vi "Analyze Data.vi"(8 "error in":errorcluster, 11 "tCRD in":refnum<class "Aircraft OPCCRD.lvclass">) -> (0 "error out":errorcluster, 3 "tCRD out":refnum<class "Aircraft OPCCRD.lvclass">)   [LabVIEW 2015, in "Aircraft OPCCRD.lvclass"]
doc: "Analyze Data takes the stored ringdown data (1000 shots per cell) and:\n1) Calculates the ringdown decay constant tau\n2) Averages tau0 data as necessary\n3) Corrects the tau data for Rayleigh scattering\n4) Stores a 1-D array of taus returned on a 1 kHz basis (8k taus) if a jump drive (U:) is connected\n5) Flattens the data into a string and stuffs the string into the <b>data</b> shared variable for display on the UI.\n\nThis VI will not be called if the data is not \"good\" (that is, if an error was thrown in the <B>Get Data</B> routine. If an error is thrown while the data is being retrieved, then the data will not be sent to the UI."
uses:
  Aircraft OPCCRD.lvclass
  Reusable/CRDS/Main/CRDS.lvclass/CRDS.ctl
  Reusable/Instrument/Instrument.lvclass/Instrument.ctl
  Aircraft OPCCRD.lvclass/Aircraft OPCCRD.ctl
  Reusable/CRDS/Cell/CRDS Cell.lvclass/CRDS Cell.ctl
  Reusable/CRDS/Data/Cell/CRDS Cell Data.lvclass/CRDS Cell Data.ctl
  <vilib>/Analysis/baseanly.llb/Matrix Type of Inverse Matrix.ctl
  Reusable/File IO/Class/File Observer.lvclass/File Observer.ctl
  <vilib>/Analysis/7linalg.llb/Solve Linear Equations (single right hand).vi
  <vilib>/Analysis/baseanly.llb/Mean (DBL).vi
  Reusable/File IO/Class/Read File Ref.vi
  Reusable/CRDS/Data/Cell/Read extParam.vi
  Reusable/CRDS/Data/Cell/Write FitCoeff.vi
  Reusable/CRDS/Data/Cell/Write extParam.vi
  Reusable/CRDS/Cell/Write Data.vi
  Accessors/Write tau Obs.vi
  Reusable/CRDS/Main/Read Laser Data.vi
  Reusable/Instrument/Read Log Session.vi
  Reusable/CRDS/Main/Read CRD RD Data Obs.vi
  Reusable/CRDS/Main/Write CRD RD Data Obs.vi
  Reusable/CRDS/Main/Read writeRDs.vi
  <vilib>/Analysis/baseanly.llb/Solve Linear Equations By Cholesky.vi
  <vilib>/Analysis/baseanly.llb/Real Matrix to Compact Array.vi
  <vilib>/Analysis/baseanly.llb/Real Compact Tri-Matrix Linear Eqs.vi
  Reusable/CRDS/Main/Read Cells.vi
  Reusable/CRDS/Main/Read goodData.vi
  Reusable/CRDS/Data/Main/Read filter.vi
  Reusable/Data/Read measTime.vi
  Reusable/CRDS/Cell/Read dt.vi
  <vilib>/Analysis/7linalg.llb/Solve Linear Eqs (General).vi
  <vilib>/Analysis/7linalg.llb/Solve Linear Eqs (Gen, single right hand).vi
  Reusable/CRDS/Data/Cell/Write Ringdowns.vi
  Reusable/CRDS/Main/Write Cells.vi
  Reusable/CRDS/Main/Write Data.vi
  Reusable/CRDS/Cell/CRDS Cell.lvclass
  Reusable/CRDS/Data/Main/CRDS Data.lvclass
  <userlib>/_Session Fwk/Session - Root.lvclass
  Reusable/CRDS/Data/Cell/CRDS Cell Data.lvclass
  Reusable/File IO/Class/File Observer.lvclass
  <vilib>/Analysis/NI_AALPro.lvlib
  <vilib>/Analysis/NI_AALBase.lvlib
  Reusable/Session Log/System Log.lvclass
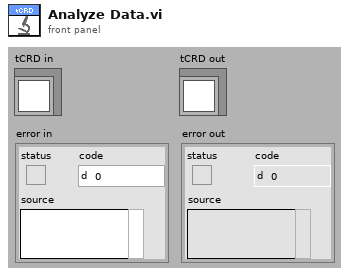
[diagram p1: front panel]
types:
  T1 = typedef "NI_AALBase.lvlib/Matrix Type of Inverse Matrix.ctl" = enum32{"General", "Positive Definite", "Lower Triangular", "Upper Triangular"}
  T2 = typedef "Session - Root.lvclass/Session Handle.ctl" = refnum<data-value>
  T3 = typedef "extparam.ctl" = cluster{"Tau":sgl, "Tau0cor":sgl, "ext":sgl, "extCorr":sgl, "stdevTau":sgl, "eTau":sgl, "taucorr":sgl, "Tau0":sgl, "max":sgl}
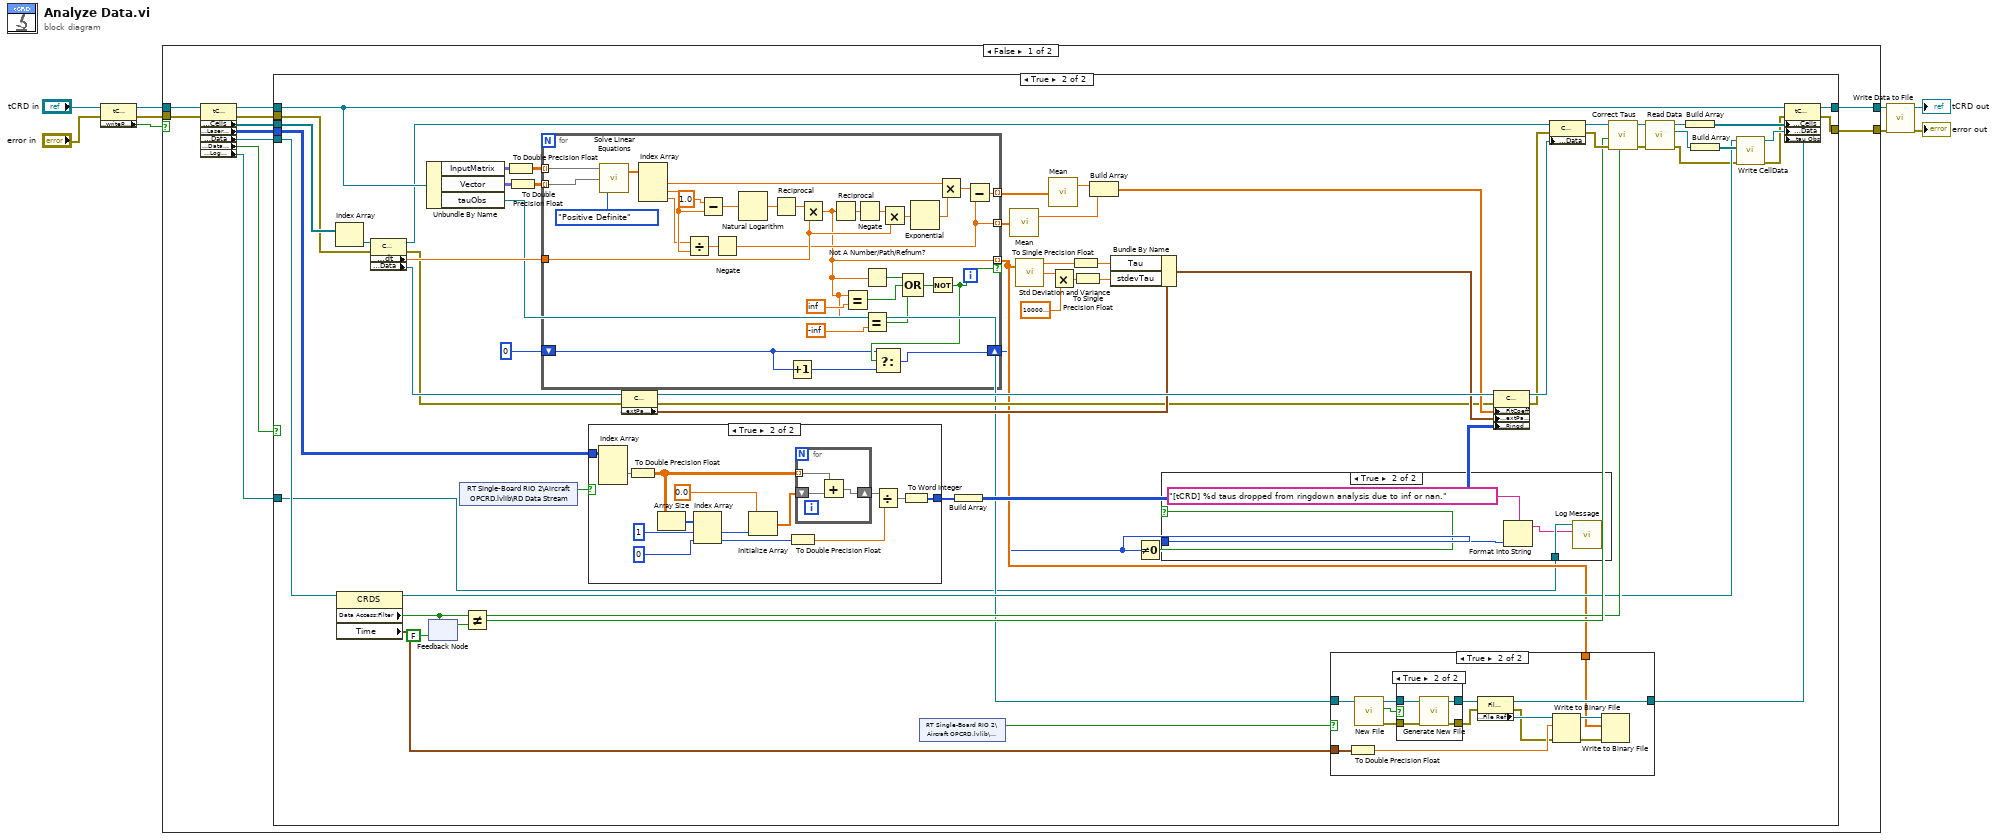
[diagram p0: block diagram]
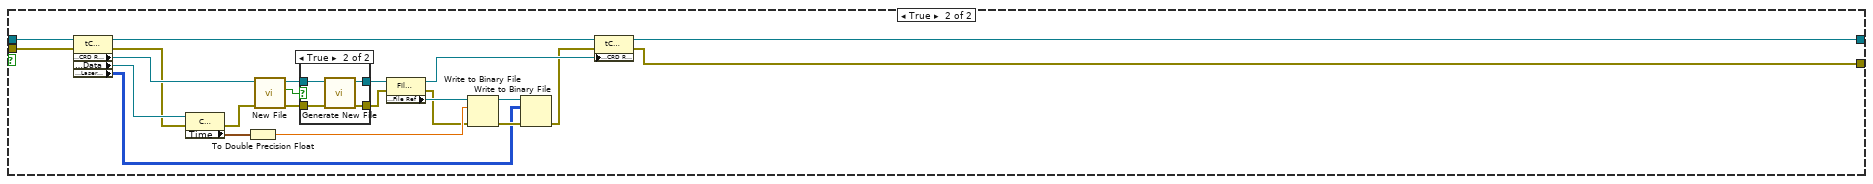
[diagram p7: hidden frame]
diagram:
  n1 = property class="tCRD"(reference="tCRD in", error in="error in") -> (reference out=w4:refnum<class "Aircraft OPCCRD.lvclass">, error out=w3:errorcluster, "Accessors:writeRDs"=w1:bool)
  n2 = case shown="False" w1 {
    tunnel: w3 -> [w20 w176]
    tunnel: [w18 w179] -> w9
    tunnel: [w17 w178] -> w7
    tunnel: w4 -> [w16 w177]
    frame False {
      n3 = property class="tCRD"(reference=w16, error in=w20) -> (reference out=w15:refnum<class "Aircraft OPCCRD.lvclass">, error out=w11:errorcluster, "Data Access:Cells"=w19:refnum<class "CRDS Cell.lvclass">[], "Data Access:Laser Data"=w13:i16[][][], "Data Access:Data"=w14:refnum<class "CRDS Data.lvclass">, "Data Access:Data Ready?"=w12:bool, "Accessors:Log Session"=w10:T2)
      n4 = case shown="True" w12 {
        tunnel: w19 -> [_ w83]
        tunnel: [w22 w63] -> w18
        tunnel: [w21 w62] -> w17
        tunnel: w15 -> [w22 w48]
        tunnel: w14 -> [_ w47]
        tunnel: w13 -> [_ w38]
        tunnel: w11 -> [w21 w34]
        tunnel: w10 -> [_ w23]
        frame False {
        }
        frame True {
          n5 = Index Array(array=w83) -> (element=w76:refnum<class "CRDS Cell.lvclass">)  [unwired: 1 in]
          n6 = property class="CRDS"(reference=w47) -> (reference out=w46:refnum<class "CRDS Data.lvclass">, "Data Access:Filter"=w70:bool, "Time"=w29:timestamp)  [unwired: 1 in, 1 out]
          n7 = property class="CRDS Cell"(reference=w76, error in=w34) -> (reference out=w45:refnum<class "CRDS Cell.lvclass">, error out=w33:errorcluster, "Data Access:dt"=w64:dbl, "Data Access:Data"=w82:refnum<class "CRDS Cell Data.lvclass">)
          n8 = Unbundle By Name(w48) -> ("InputMatrix"=w61:fxp<+/-,64,64>[][][], "Vector"=w59:fxp<+/-,64,64>[][], "tauObs"=w31:refnum<class "File Observer.lvclass">)
          n9 = feedback #1(FALSE ("filter")) -> (w56:bool)
          n10 = feedback-in #1(w70) -> ()
          n11 = shared-variable "RT Single-Board RIO 2\\Aircraft OPCRD.lvlib\\RD Data Stream"() -> (w49:bool)  [unwired: 1 in, 1 out]
          n12 = Not Equal?(x=w70, y=w56) -> (x != y?=w71:bool)
          n13 = To Double Precision Float(number=w61) -> (double precision float=w60:dbl[][][])
          n14 = To Double Precision Float(number=w59) -> (double precision float=w58:dbl[][])
          n15 = for {
            tunnel: w58 -> [w141] mode=indexing
            tunnel: w64 -> [w140]
            tunnel: [w134] -> w28 mode=indexing if=w129
            tunnel: w60 -> [w139] mode=indexing
            tunnel: [w138] -> w54 mode=indexing
            tunnel: [w137] -> w53 mode=indexing
            shift-right: [w126] -> w25
            shift-left: 0 -> [w128]
            n16 = call-poly <vilib>:"Solve Linear Equations.vi"("matrix type"=Matrix_Type_of_Inverse_Matrix."Positive Definite", "Known Vector"=w141, "Input Matrix"=w139) -> ("Solution Vector"=w155:dbl[])  [unwired: 1 out]
            n17 = Index Array(array=w155) -> (element #1=w144:dbl, element #2=w143:dbl, element #3=w142:dbl)  [unwired: 3 in]
            n18 = Divide(x=w142, y=w143) -> (x/y=w150:dbl)
            n19 = Subtract(x=1.0, y=w143) -> (x-y=w153:dbl)
            n20 = Negate(x=w150) -> (-x=w138:dbl)
            n21 = Natural Logarithm(1:w153) -> (0:w152:dbl)
            n22 = Reciprocal(x=w152) -> (1/x=w151:dbl)
            n23 = Increment(x=w128) -> (x+1=w127:i32)
            n24 = Multiply(x=w151, y=w140) -> (x*y=w134:dbl)
            n25 = Reciprocal ("beta")(x=w134) -> (1/x=w149:dbl)
            n26 = Equal?(x=w134, y=inf) -> (x = y?=w132:bool)
            n27 = Negate(x=w149) -> (-x=w148:dbl)
            n28 = Not A Number/Path/Refnum?(number/path/refnum=w134) -> (NaN/Path/Refnum?=w133:bool)
            n29 = Equal?(x=w134, y=-inf) -> (x = y?=w130:bool)
            n30 = Multiply(x=w148, y=w140) -> (x*y=w147:dbl)
            n31 = Compound Arithmetic op=OR(w133, w132, w130) -> (w131:bool)
            n32 = Exponential(1:w147) -> (0:w145:dbl)
            n33 = Not(x=w131) -> (.not. x?=w129:bool)
            n34 = Select(t=w128, s=w129, f=w127) -> (s? t:f=w126:i32)
            n35 = Multiply(x=w144, y=w145) -> (x*y=w146:dbl)
            n36 = Subtract(x=w146, y=w138) -> (x-y=w137:dbl)
          }
          n37 = case shown="True" w49 {
            tunnel: [_ w121] -> w57
            tunnel: w38 -> [_ w115]
            frame False {
            }
            frame True {
              n38 = Index Array(array=w115) -> (element=w119:i16[][])  [unwired: 3 in]
              n39 = To Double Precision Float(number=w119) -> (double precision float=w113:dbl[][])
              n40 = Array Size(array=w113) -> (size(s)=w116:i32[])
              n41 = Index Array(array=w116, index #1=1 ("index"), index #2=0 ("index")) -> (element #1=w118:i32, element #2=w109:i32)
              n42 = Initialize Array(0.0 ("element"), w118) -> (w114:dbl[])
              n43 = To Double Precision Float(number=w109) -> (double precision float=w112:dbl)
              n44 = for {
                shift-right: [w123] -> w120
                shift-left: w114 -> [w124]
                tunnel: w113 -> [w125] mode=indexing
                n45 = Add(x=w125, y=w124) -> (x+y=w123:dbl[])
              }
              n46 = Divide(x=w120, y=w112) -> (x/y=w122:dbl[])
              n47 = To Word Integer(number=w122) -> (16bit integer=w121:i16[])
            }
          }
          n48 = property class="CRDS Cell"(reference=w82, error in=w33) -> (reference out=w81:refnum<class "CRDS Cell Data.lvclass">, error out=w32:errorcluster, "Data Access:extParam"=w80:T3)
          n49 = shared-variable "RT Single-Board RIO 2\\Aircraft OPCRD.lvlib\\WriteTau"() -> (w27:bool)  [unwired: 1 in, 1 out]
          n50 = Build Array(w57) -> (w79:i16[][])
          n51 = call-poly <vilib>:"Mean.vi"("X"=w54) -> ("mean"=w51:dbl)  [unwired: 1 out]
          n52 = call <vilib>:"Std Deviation and Variance.vi"("X"=w28) -> ("mean"=w42:dbl, "standard deviation"=w78:dbl)  [unwired: 1 in, 1 out]
          n53 = call-poly <vilib>:"Mean.vi"("X"=w53) -> ("mean"=w52:dbl)  [unwired: 1 out]
          n54 = Multiply(x=w78, y=1000000.0 ("stdevTau")) -> (x*y=w44:dbl)
          n55 = To Single Precision Float(number=w42) -> (single precision float=w41:sgl)
          n56 = To Single Precision Float(number=w44) -> (single precision float=w43:sgl)
          n57 = Build Array(w52, w51) -> (w39:dbl[])
          n58 = Bundle By Name(cluster=w80, "Tau"=w41, "stdevTau"=w43) -> (w40:T3)
          n59 = Not Equal To 0?(x=w25) -> (x != 0?=w24:bool)
          n60 = case shown="True" w24 {
            tunnel: w25 -> [_ w87]
            tunnel: w23 -> [_ w86]
            frame False {
            }
            frame True {
              n61 = Format Into String(format string="[tCRD] %d taus dropped from ringdown analysis due to inf or nan.", w87) -> (resulting string=w85:string)  [unwired: 2 in, 1 out]
              n62 = call "Log Message.vi"("MSG In"=w85, "session in"=w86) -> ()  [unwired: 8 in, 2 out]
            }
          }
          n63 = case shown="True" w27 {
            tunnel: w31 -> [w88 w92]
            tunnel: [w88 w91] -> w30
            tunnel: w29 -> [_ w90]
            tunnel: w28 -> [_ w89]
            frame False {
            }
            frame True {
              n64 = To Double Precision Float(number=w90) -> (double precision float=w96:dbl)
              n65 = call-dynamic "New File.vi"("File Observer in"=w92) -> ("error out"=w102:errorcluster, "Exceeded"=w101:bool, "File Observer out"=w100:refnum<class "File Observer.lvclass">)  [unwired: 8 in]
              n66 = case shown="True" w101 {
                tunnel: w100 -> [w104 w108]
                tunnel: [w104 w107] -> w99
                tunnel: w102 -> [w103 w106]
                tunnel: [w103 w105] -> w94
                frame False {
                }
                frame True {
                  n67 = call-dynamic "Generate New File.vi"("error in"=w106, "File Obs in"=w108) -> ("error out"=w105:errorcluster, "File Obs out"=w107:refnum<class "File Observer.lvclass">)  [unwired: 7 in, 1 out]
                }
              }
              n68 = property class="File Obs"(reference=w99, error in=w94) -> (reference out=w91:refnum<class "File Observer.lvclass">, error out=w93:errorcluster, "Data Access:File Ref"=w98:refnum<file>)
              n69 = Write to Binary File(file (use dialog)=w98, data=w96, error in=w93) -> (refnum out=w97:refnum<file>, error out=w95:errorcluster)  [unwired: 3 in, 1 out]
              n70 = Write to Binary File(file (use dialog)=w97, data=w89, error in=w95) -> ()  [unwired: 3 in, 3 out]
            }
          }
          n71 = property class="CRDS Cell"(reference=w81, error in=w32, "Accessors:FitCoeff"=w39, "Data Access:extParam"=w40, "Data Access:Ringdowns"=w79) -> (reference out=w50:refnum<class "CRDS Cell Data.lvclass">, error out=w37:errorcluster)
          n72 = property class="CRDS Cell"(reference=w45, error in=w37, "Data Access:Data"=w50) -> (reference out=w75:refnum<class "CRDS Cell.lvclass">, error out=w74:errorcluster)
          n73 = call "Correct Taus.vi"("Filter?"=w70, "error in"=w74, "filter changed?"=w71, "CRDS Cell in"=w75) -> ("error out"=w72:errorcluster, "CRDS Cell out"=w73:refnum<class "CRDS Cell.lvclass">)  [unwired: 6 in]
          n74 = call "Read Data.vi"("error in"=w72, "CRDS Cell in"=w73) -> ("error out"=w36:errorcluster, "CRDS Cell"=w65:refnum<class "CRDS Cell Data.lvclass">, "CRDS Cell out"=w68:refnum<class "CRDS Cell.lvclass">)  [unwired: 7 in]
          n75 = Build Array(w68) -> (w67:refnum<class "CRDS Cell.lvclass">[])
          n76 = Build Array(w65) -> (w69:refnum<class "CRDS Cell Data.lvclass">[])
          n77 = call "Write CellData.vi"("error in"=w36, "CellData"=w69, "CRDS Data in"=w46) -> ("error out"=w35:errorcluster, "CRDS Data out"=w66:refnum<class "CRDS Data.lvclass">)  [unwired: 7 in]
          n78 = property class="tCRD"(reference=w48, error in=w35, "Data Access:Cells"=w67, "Data Access:Data"=w66, "Accessors:tau Obs"=w30) -> (reference out=w63:refnum<class "Aircraft OPCCRD.lvclass">, error out=w62:errorcluster)
        }
      }
    }
    frame True {
      n79 = property class="tCRD"(reference=w177, error in=w176) -> (reference out=w157:refnum<class "Aircraft OPCCRD.lvclass">, error out=w161:errorcluster, "Accessors:CRD RD Data Obs"=w162:refnum<class "File Observer.lvclass">, "Data Access:Data"=w163:refnum<class "CRDS Data.lvclass">, "Data Access:Laser Data"=w160:i16[][][])
      n80 = property class="CRDS"(reference=w163, error in=w161) -> (error out=w164:errorcluster, "Time"=w169:timestamp)  [unwired: 1 out]
      n81 = To Double Precision Float(number=w169) -> (double precision float=w168:dbl)
      n82 = call-dynamic "New File.vi"("error in"=w164, "File Observer in"=w162) -> ("error out"=w175:errorcluster, "Exceeded"=w174:bool, "File Observer out"=w173:refnum<class "File Observer.lvclass">)  [unwired: 7 in]
      n83 = case shown="True" w174 {
        tunnel: w173 -> [w181 w185]
        tunnel: [w181 w184] -> w172
        tunnel: w175 -> [w180 w183]
        tunnel: [w180 w182] -> w166
        frame False {
        }
        frame True {
          n84 = call-dynamic "Generate New File.vi"("error in"=w183, "File Obs in"=w185) -> ("error out"=w182:errorcluster, "File Obs out"=w184:refnum<class "File Observer.lvclass">)  [unwired: 7 in, 1 out]
        }
      }
      n85 = property class="File Obs"(reference=w172, error in=w166) -> (reference out=w159:refnum<class "File Observer.lvclass">, error out=w165:errorcluster, "Data Access:File Ref"=w171:refnum<file>)
      n86 = Write to Binary File(file (use dialog)=w171, data=w168, error in=w165) -> (refnum out=w170:refnum<file>, error out=w167:errorcluster)  [unwired: 3 in, 1 out]
      n87 = Write to Binary File(file (use dialog)=w170, data=w160, error in=w167) -> (error out=w158:errorcluster)  [unwired: 3 in, 2 out]
      n88 = property class="tCRD"(reference=w157, error in=w158, "Accessors:CRD RD Data Obs"=w159) -> (reference out=w179:refnum<class "Aircraft OPCCRD.lvclass">, error out=w178:errorcluster)
    }
  }
  n89 = call-dynamic "Write Data to File.vi"("error in"=w7, "tCRD in"=w9) -> ("error out"=→"error out":errorcluster, "tCRD out"=→"tCRD out":refnum<class "Aircraft OPCCRD.lvclass">)  [unwired: 8 in]
